vi "3.2.vi"() -> ()   [LabVIEW 2014]
panel:
  out "Number Of Iterations":dbl
  out "Current Number":dbl
  in  "Number To Match":dbl
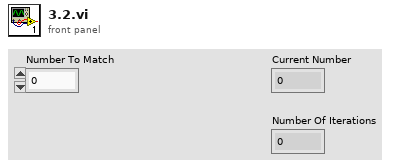
[diagram p1: front panel]
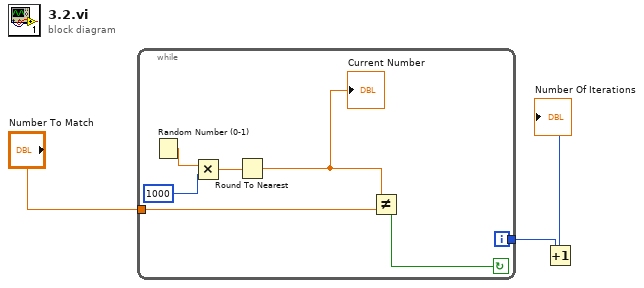
[diagram p0: block diagram]
diagram:
  n1 = while {
    tunnel: "Number To Match" -> [w8]
    tunnel: [w4] -> w2
    i -> [w4]
    stop <- w5 continue-if-true
    n2 = Random Number (0-1)() -> (number: 0 to 1=w6:dbl)
    n3 = Multiply(x=w6, y=1000) -> (x*y=w10:dbl)
    n4 = Round To Nearest(number=w10) -> (nearest integer value=w9:dbl)
    "Current Number" <- w9
    n5 = Not Equal?(x=w9, y=w8) -> (x != y?=w5:bool)
  }
  n6 = Increment(x=w2) -> (x+1=→"Number Of Iterations":i32)
